vi "_Global variables 1.vi"() -> ()   [LabVIEW 2019]
uses:
  Controls/IPS system status_m.ctl
  Controls/IPS system status_n.ctl
  Controls/IPS activity.ctl
  Controls/IPS loc-rem status.ctl
  Controls/IPS switch heater status.ctl
  Controls/IPS mode_m.ctl
  Controls/IPS mode_n.ctl
  Controls/IPS polarity_m.ctl
  Controls/IPS polarity_n.ctl
panel:
  in  "Control channel":enum16{"Sample stage", "Mixing chamber"}(ring)=enum."Mixing chamber"
  in  "Recording channel":enum16{"Sample stage", "Mixing chamber"}(ring)
  out "Downscan command":string
  out "Upscan command":string
  in  "Lower field":dbl format="%_3g"
  in  "Upper field":dbl format="%_3g"
  in  "Temp tolerance":dbl format="%_3g"
  in  "Temp Step":dbl format="%_3g"
  in  "Final Temp":dbl format="%_3g"
  in  "Init Temp":dbl format="%_3g"
  in  "Excitation current":dbl=1e-05
  in  "Volt meter":refnum<visa-resource-name>="GPIB0::12::INSTR"
  in  "Current source":refnum<visa-resource-name>="GPIB0::12::INSTR"
  in  "Switch":refnum<visa-resource-name>="GPIB0::12::INSTR"
  in  "Data acquisition field interval (T)":dbl=0.001
  in  "Serial Resistor":dbl=51000.0
  in  "Lock-in Address":refnum<visa-resource-name>="GPIB0::12::INSTR"
  in  "IPS status":T10
  out "Status notifier":refnum<notifier>
  in  "UI log queue":refnum<queue>
  in  "IPS delay after heater is ON (s)":i32=30 min=0 max=1000
  out "Status":string
  in  "Lakeshore B channel":u8=5 min=1 max=16
  in  "Lakeshore A channel":u8=1 min=1 max=16
  in  "LakeShore B address":refnum<visa-resource-name>="GPIB0::4::INSTR"
  in  "LakeShore A address":refnum<visa-resource-name>="GPIB0::3::INSTR"
  in  "Data files directory":path=path "D:/ACM_measurements"
  out "Fieldscan is running":bool
  in  "Stop execution":bool
  in  "IPS address":refnum<visa-resource-name>="GPIB0::25::INSTR"
  in  "Batch files directory":path=path "D:/ACM in LabVIEW/_batch (NIW test)"
  in  "Log files directory":path=path "D:/ACM in LabVIEW/_LogBooks (NIW test)"
  # "LakeShore 370"
  # "IPS magnet power supply"
  # "Lock-In Amplifier 1"
  # "Van Der Paul measurement"
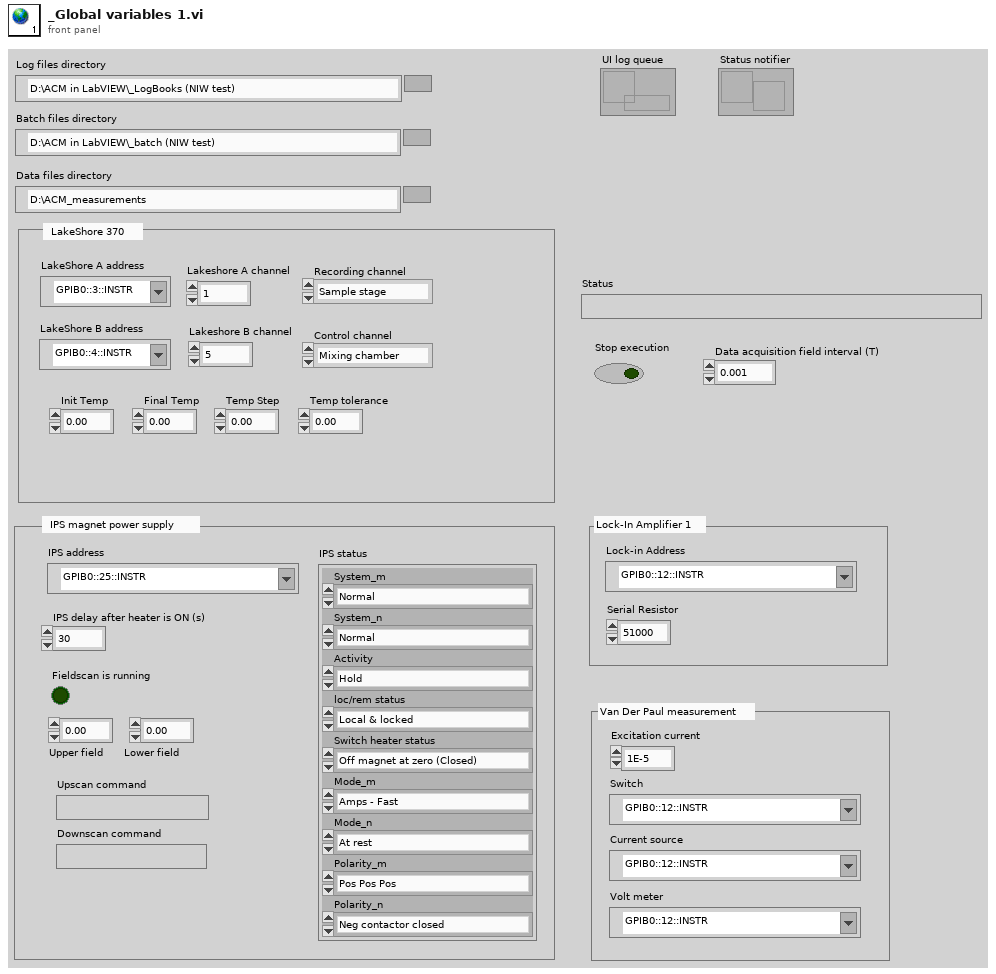
[diagram p1: front panel]
types:
  T1 = typedef "IPS system status_m.ctl" = enum16{"Normal", "Quenched", "Over heated", "_unused3", "Warming up", "_unused5", "_unused6", "_unused7", "Fault"}
  T2 = typedef "IPS system status_n.ctl" = enum16{"Normal", "On positive voltage limit", "On negative voltage limit", "_unused3", "Outside negative current limit", "_unused5", "_unused6", "_unused7", "Outside positive current limit"}
  T3 = typedef "IPS activity.ctl" = enum16{"Hold", "To setpoint", "To zero", "_unused3", "Clamped"}
  T4 = typedef "IPS loc-rem status.ctl" = enum16{"Local & locked", "Remote & locked", "Local & unlocked", "Remote & unlocked", "Auto-run-down4", "Auto-run-down5", "Auto-run-down6", "Auto-run-down7"}
  T5 = typedef "IPS switch heater status.ctl" = enum16{"Off magnet at zero (Closed)", "On (Open)", "Off magnet at field (Closed)", "_unused3", "_unused4", "Heater fault", "_unused6", "_unused7", "No switch fitted"}
  T6 = typedef "IPS mode_m.ctl" = enum16{"Amps - Fast", "Tesla - Fast", "_unused2", "_unused3", "Amps - Slow", "Tesla - Slow"}
  T7 = typedef "IPS mode_n.ctl" = enum16{"At rest", "Sweeping", "Sweep limiting", "Sweeping & sweep limiting"}
  T8 = typedef "IPS polarity_m.ctl" = enum16{"Pos Pos Pos", "Pos Pos Neg", "Pos Neg Pos", "Pos Neg Neg", "Neg Pos Pos", "Neg Pos Neg", "Neg Neg Pos", "Neg Neg Neg"}
  T9 = typedef "IPS polarity_n.ctl" = enum16{"Neg contactor closed", "Pos contactor closed", "Both contactors open", "Both contactors closed"}
  T10 = cluster{"System_m":T1, "System_n":T2, "Activity":T3, "loc/rem status":T4, "Switch heater status":T5, "Mode_m":T6, "Mode_n":T7, "Polarity_m":T8, "Polarity_n":T9}
diagram:
